vi "CCE MGLD PMJD PF SubVI05.vi"(6 "Coordenadas":T2, 9 "UMBRAL":u8(knob) scale=0.0..255.0, 10 "Tolerancia":dbl, 11 "Image":T1) -> (0 "Estado botella":string, 2 "Abolladuas?":bool)   [LabVIEW 2020]
doc: "Ceballos Conde Emanuel Meneses Gutiérrez Luis David Pineda Méndez Job Daniel 4MV6 Sistemas de visión artificial 2022/1 \nEste vi permite obtener el estado de la zona baja de una botella para determinar si presenta abolladuras o no, en necesario que la botella cuente con liquido para lograr determinar su estado"
uses:
  <vilib>/vision/Image Controls.llb/IMAQ Image.ctl
panel:
  out "Image 2":T1(plugin-control)
  out "Diferencia":dbl
  out "Memoria":picture
  out "Muestra":picture
  # "Ceballos Conde Emanuel   -  Meneses Gutiérrez Luis David   -  Pineda Méndez Job Daniel 4MV6 Sistemas de visión artificial  2022/1             SubVI05"
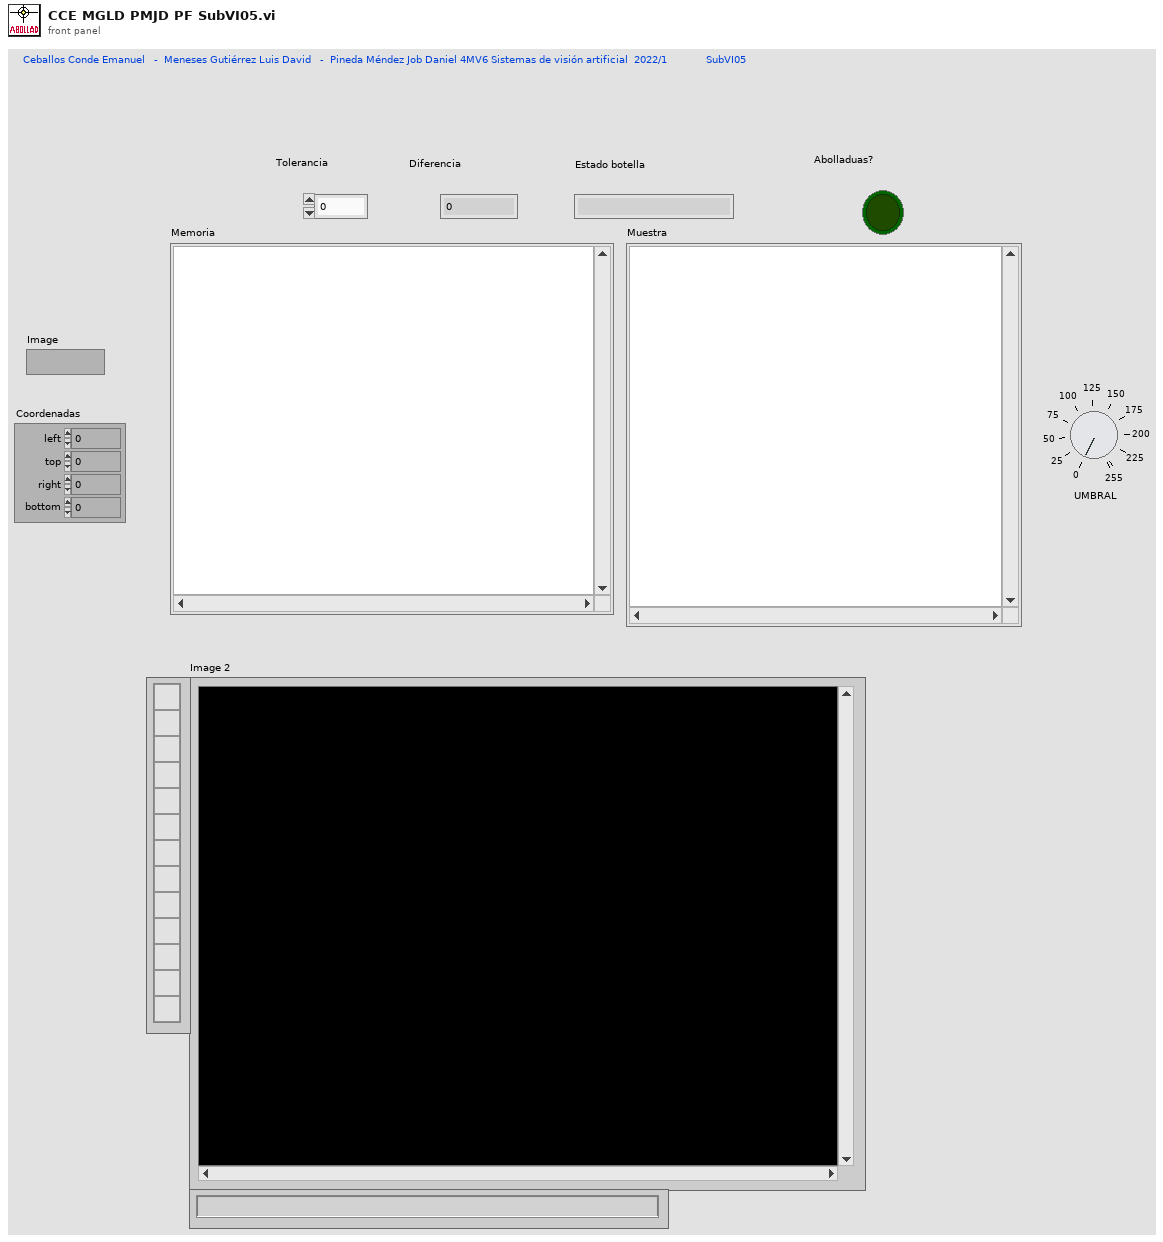
[diagram p1: front panel]
types:
  T1 = typedef "IMAQ Image.ctl" = refnum<image>
  T2 = cluster{"left":i16, "top":i16, "right":i16, "bottom":i16}
  T3 = typedef "Image Type" = u32
  T4 = typedef "imagedata.ctl" = cluster{"image type":i32, "image depth":i32, "image":u8[], "mask":u8[], "colors":u32[], "Rectangle":cluster{"left":i16, "top":i16, "right":i16, "bottom":i16}}
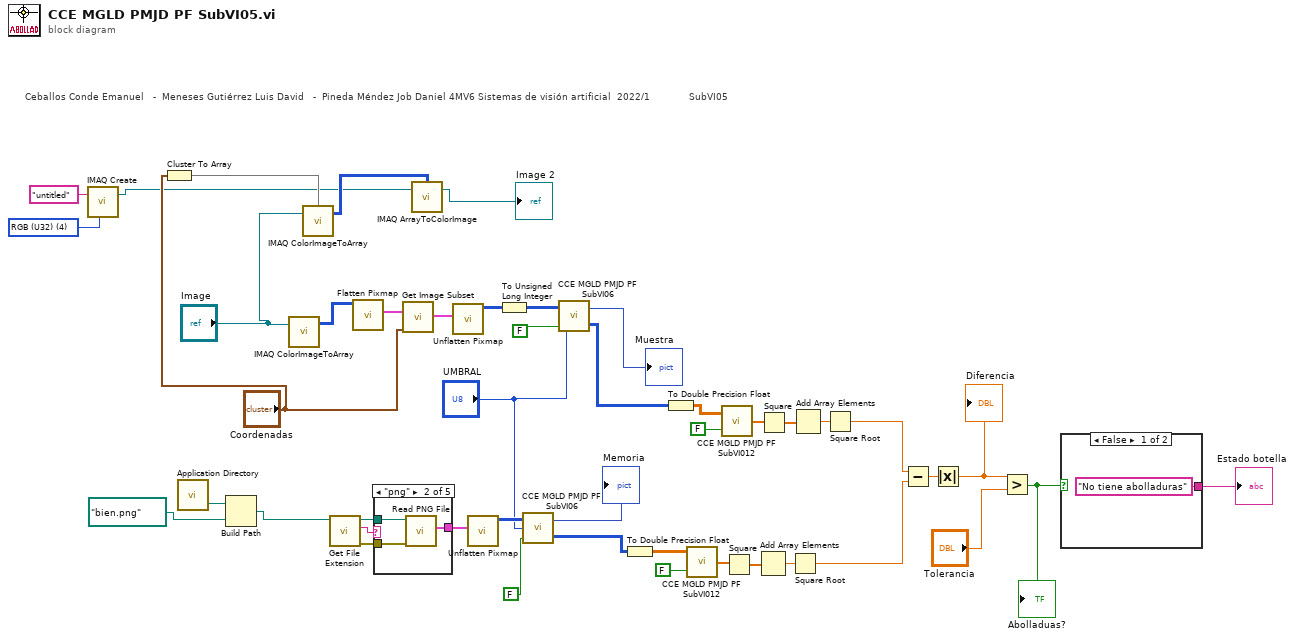
[diagram p0: block diagram]
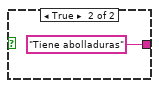
[diagram p2: hidden frame]
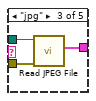
[diagram p4: hidden frame]
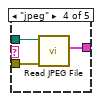
[diagram p5: hidden frame]
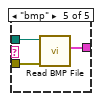
[diagram p6: hidden frame]
diagram:
  w4 = T3 4 items=["Grayscale (U8)", "Grayscale (I16)", "Grayscale (SGL)", "Complex (CSG)", "RGB (U32)", "HSL (U32)", "RGB (U64)", "Grayscale (U16)"] ("Image Type")
  # "Ceballos Conde Emanuel   -  Meneses Gutiérrez Luis David   -  Pineda Méndez Job Daniel 4MV6 Sistemas de visión artificial  2022/1             SubVI05"
  n1 = call "IMAQ Create"("Image Name"="untitled", "Image Type"=w4) -> ("New Image"=w6:T1)  [unwired: 3 in, 1 out]
  n2 = Cluster To Array(cluster="Coordenadas") -> (array=w8:i16[])
  n3 = call <vilib>:"Application Directory.vi"() -> ("Application Directory"=w3:path)
  n4 = Build Path(base path=w3, name or relative path=path "bien.png") -> (appended path=w1:path)
  n5 = call "IMAQ ColorImageToArray"("Image"="Image") -> ("Image Pixels (U32)"=w13:u32[][])  [unwired: 3 in, 2 out]
  n6 = call "IMAQ ColorImageToArray"("Optional Rectangle"=w8, "Image"="Image") -> ("Image Pixels (U32)"=w10:u32[][])  [unwired: 2 in, 2 out]
  n7 = call <vilib>:"Get File Extension.vi"("file"=w1) -> ("error out"=w41:errorcluster, "lowercase file extension"=w43:string, "dup file"=w42:path)  [unwired: 6 in, 2 out]
  n8 = call <vilib>:"Flatten Pixmap.vi"("24-bit pixmap"=w13) -> ("image data"=w16:T4)  [unwired: 10 in]
  n9 = case shown="\"png\"" w43 {
    tunnel: w42 -> [_ w48 w49 w54 w56]
    tunnel: w41 -> [_ w47 w51 w53 w57]
    tunnel: [_ w46 w50 w52 w55] -> w40
    frame "False", Default {
    }
    frame "png" {
      n10 = call <vilib>:"Read PNG File.vi"("error in (no error)"=w47, "path to PNG file"=w48) -> ("image data"=w46:T4)  [unwired: 7 in, 2 out]
    }
    frame "jpg" {
      n11 = call <vilib>:"Read JPEG File.vi"("error in (no error)"=w51, "path to JPEG file"=w49) -> ("image data"=w50:T4)  [unwired: 7 in, 2 out]
    }
    frame "jpeg" {
      n12 = call <vilib>:"Read JPEG File.vi"("error in (no error)"=w53, "path to JPEG file"=w54) -> ("image data"=w52:T4)  [unwired: 7 in, 2 out]
    }
    frame "bmp" {
      n13 = call <vilib>:"Read BMP File.vi"("error in (no error)"=w57, "path to BMP file"=w56) -> ("image data"=w55:T4)  [unwired: 7 in, 2 out]
    }
  }
  n14 = call <vilib>:"Get Image Subset.vi"("subset rect"="Coordenadas", "image data"=w16) -> ("image subset"=w15:T4)  [unwired: 4 in, 1 out]
  n15 = call "IMAQ ArrayToColorImage"("Image Pixels (U32)"=w10, "Image"=w6) -> ("Image Out"=→"Image 2":T1)  [unwired: 3 in, 1 out]
  n16 = call <vilib>:"Unflatten Pixmap.vi"("image data"=w15) -> ("24-bit pixmap"=w14:u32[][])  [unwired: 4 in, 6 out]
  n17 = call <vilib>:"Unflatten Pixmap.vi"("image data"=w40) -> ("24-bit pixmap"=w38:u32[][])  [unwired: 4 in, 6 out]
  n18 = To Unsigned Long Integer(number=w14) -> (unsigned 32bit integer=w17:u32[][])
  n19 = call "CCE MGLD PMJD PF SubVI06.vi"("INVERTIDO?"=FALSE, "UMBRAL"="UMBRAL", "pixmap"=w38) -> ("Umbralizado"=w18:u8[][], "IMG"=→"Memoria":picture)
  n20 = call "CCE MGLD PMJD PF SubVI06.vi"("INVERTIDO?"=FALSE, "UMBRAL"="UMBRAL", "pixmap"=w17) -> ("Umbralizado"=w20:u8[][], "IMG"=→"Muestra":picture)
  n21 = To Double Precision Float(number=w18) -> (double precision float=w19:dbl[][])
  n22 = To Double Precision Float(number=w20) -> (double precision float=w21:dbl[][])
  n23 = call "CCE MGLD PMJD PF SubVI012.vi"("NORMALIZACIÓN"=FALSE, "f"=w19) -> ("MOMENTOS Hu"=w36:dbl[])
  n24 = call "CCE MGLD PMJD PF SubVI012.vi"("NORMALIZACIÓN"=FALSE, "f"=w21) -> ("MOMENTOS Hu"=w31:dbl[])
  n25 = Square(x=w36) -> (x^2=w35:dbl[])
  n26 = Add Array Elements(numeric array=w35) -> (sum=w34:dbl)
  n27 = Square(x=w31) -> (x^2=w33:dbl[])
  n28 = Square Root(x=w34) -> (sqrt(x)=w29:dbl)
  n29 = Add Array Elements(numeric array=w33) -> (sum=w32:dbl)
  n30 = Square Root(x=w32) -> (sqrt(x)=w30:dbl)
  n31 = Subtract(x=w30, y=w29) -> (x-y=w28:dbl)
  n32 = Absolute Value(x=w28) -> (abs(x)=w27:dbl)
  "Diferencia" <- w27
  n33 = Greater?(x=w27, y="Tolerancia") -> (0:w26:bool)
  "Abolladuas?" <- w26
  n34 = case shown="False" w26 {
    tunnel: ["No tiene abolladuras" "Tiene abolladuras"] -> w25
    frame False {
    }
    frame True {
    }
  }
  "Estado botella" <- w25
